vi "Logger_Exit.vi"(8 "error in (no error)":errorcluster caption="错误输入（无错误）") -> (0 "error out":errorcluster caption="错误输出")   [LabVIEW 2019, in "Logger.lvclass"]
uses:
  <userlib>/Logger/Logger.lvclass
  <userlib>/Logger/Ctls/LoggerMessage.ctl
  <userlib>/Logger/Logger.lvclass/Logger.ctl
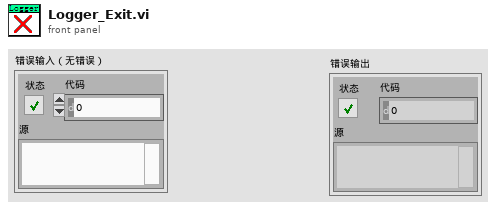
[diagram p1: front panel]
types:
  T1 = typedef "Logger.lvclass/LoggerMessage.ctl" = cluster{"LoggerKind":enum16{"软件上传日志", "软件其他日志", "软件错误日志", "软件监控日志"}, "LoggerMessage":string, "LoggerCode":i32, "LoggerCallChain":string, "LoggerTime":string}
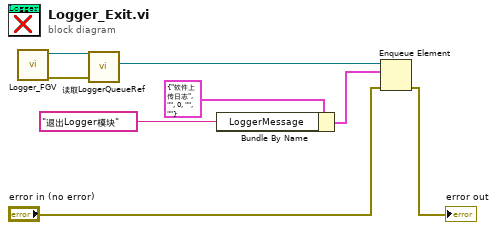
[diagram p0: block diagram]
diagram:
  n1 = call <userlib>:"Logger_FGV.vi"() -> ("error out"=w7:errorcluster, "Logger 输出"=w8:refnum<class "Logger.lvclass">)  [unwired: 10 in]
  n2 = call "读取LoggerQueueRef.vi"("error in (no error)"=w7, "Logger输入"=w8) -> ("LoggerQueueRef"=w6:refnum<queue>)  [unwired: 7 in, 2 out]
  n3 = Bundle By Name(cluster=T1 {"LoggerKind"=enum."软件上传日志", "LoggerMessage"="", "LoggerCode"=0, "LoggerCallChain"="", "LoggerTime"=""} ("元素"), "LoggerMessage"="退出Logger模块" ("source")) -> (w3:T1)
  n4 = Enqueue Element(queue=w6, element=w3, error in (no error)="error in (no error)") -> (error out=→"error out":errorcluster)  [unwired: 1 in, 2 out]
